vi "StringIOArray.vi"() -> ()   [LabVIEW 2015]
panel:
  out "error out":errorcluster
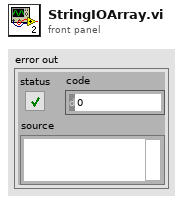
[diagram p1: front panel]
types:
  T1 = enum16{"open", "replace", "create", "open or create", "replace or create", "replace or create with confirmation"}
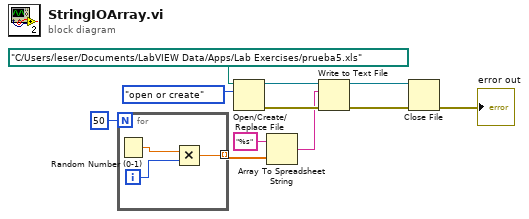
[diagram p0: block diagram]
diagram:
  n1 = for {
    N: 50 -> [_]
    tunnel: [w12] -> w9 mode=indexing
    i -> [w13]
    n2 = Random Number (0-1)() -> (number: 0 to 1=w14:dbl)
    n3 = Multiply(x=w14, y=w13) -> (x*y=w12:dbl)
  }
  n4 = Open/Create/Replace File(file path (use dialog)=path "C:/Users/leser/Documents/LabVIEW Data/Apps/Lab Exercises/prueba5.xls", operation (0:open)=T1."open or create") -> (refnum out=w5:refnum<file>, error out=w6:errorcluster)  [unwired: 4 in, 1 out]
  n5 = Array To Spreadsheet String(array=w9, 3:"%s" ("format string")) -> (spreadsheet string=w4:string)  [unwired: 1 in]
  n6 = Write to Text File(file (use dialog)=w5, text=w4, error in=w6) -> (refnum out=w3:refnum<file>, error out=w2:errorcluster)  [unwired: 1 in, 1 out]
  n7 = Close File(refnum=w3, error in=w2) -> (error out=→"error out":errorcluster)  [unwired: 1 out]
